vi "GoTo.vi"(6 "Busy":refnum<vi>, 8 "error in (no error)":errorcluster, 10 "Param":string, 11 "Controlador in":refnum<class "Controlador.lvclass">) -> (0 "error out":errorcluster, 2 "Response":string, 3 "Controlador out":refnum<class "Controlador.lvclass">)   [LabVIEW 2011]
uses:
  GLOBAL.vi
  Controlador.lvclass
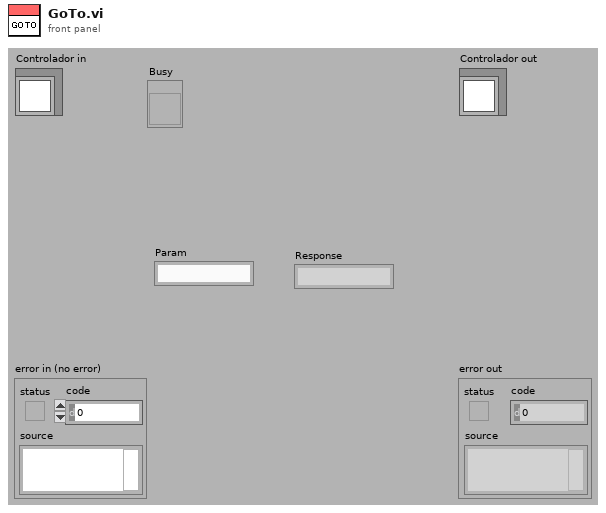
[diagram p1: front panel]
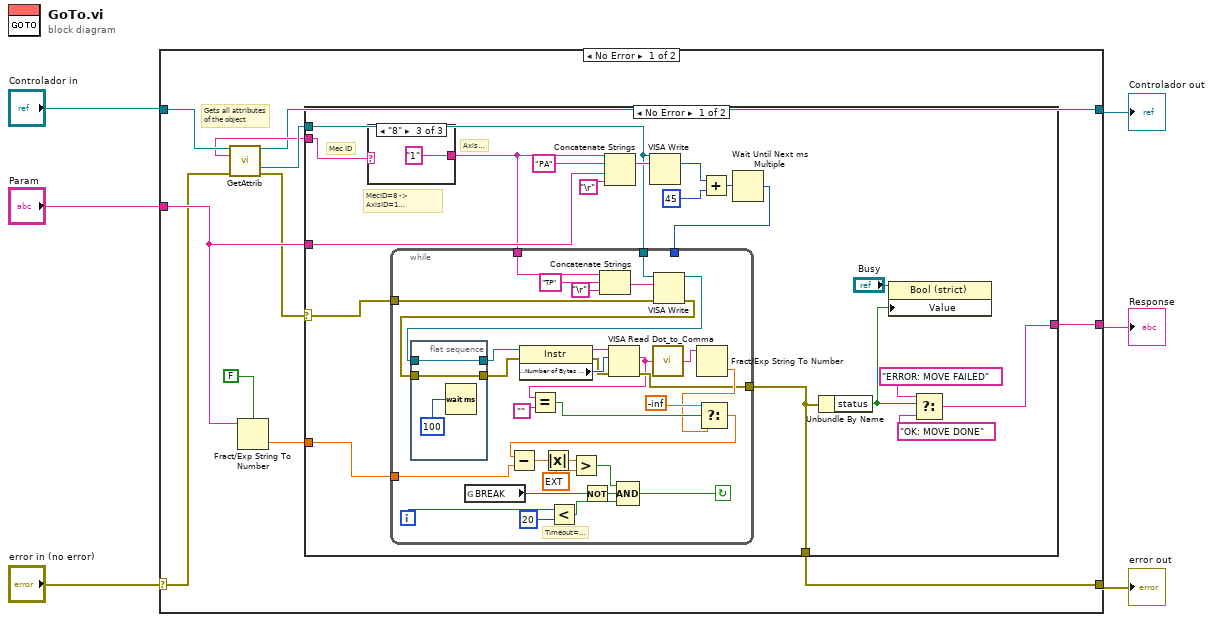
[diagram p0: block diagram]
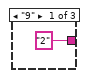
[diagram p2: hidden frame]
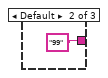
[diagram p3: hidden frame]
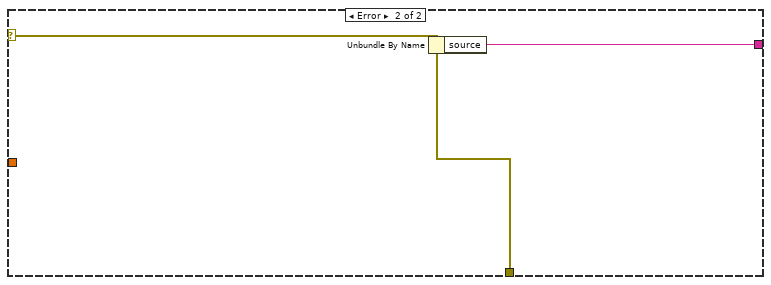
[diagram p4: hidden frame]
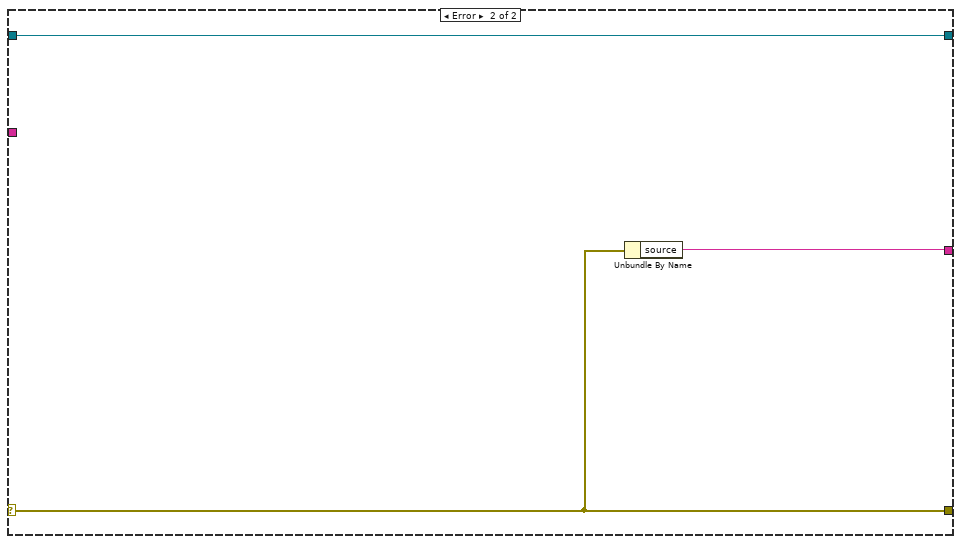
[diagram p5: hidden frame]
diagram:
  n1 = case shown="No Error" "error in (no error)" {
    selector: "error in (no error)" -> [w15 w78]
    tunnel: [w11 w79] -> w6
    tunnel: "Controlador in" -> [w14 w79]
    tunnel: [w10 w78] -> w2
    tunnel: "Param" -> [w17 _]
    tunnel: [w9 w77] -> w1
    frame No Error {
      # "Gets all attributes \nof the object"
      n2 = call "GetAttrib.vi"("Device in"=w14, "error in (no error)"=w15) -> ("Device out"=w11:refnum<class "Controlador.lvclass">, "Mec ID"=w12:string, "VISA Mec"=w13:refnum<visa-resource-name>, "error out"=w8:errorcluster)  [unwired: 10 out]
      n3 = Fract/Exp String To Number(use system decimal point (T)=FALSE, string=w17) -> (number=w16:dbl)  [unwired: 3 out]
      n4 = case shown="No Error" w8 {
        selector: w8 -> [w22 w76]
        tunnel: w17 -> [w29 _]
        tunnel: w16 -> [w28 _]
        tunnel: w13 -> [w27 _]
        tunnel: w12 -> [w18 _]
        tunnel: [w26 w76] -> w10
        tunnel: [w23 w75] -> w9
        frame No Error {
          # "MecID=8 -> AxisID=1\nMecID=9 -> AxisID=2"
          # "Axis ID"
          # "Mec ID"
          n5 = case shown="\"8\"" w18 {
            tunnel: ["2" "99" "1"] -> w19
            frame "9" {
            }
            frame Default {
            }
            frame "8" {
            }
          }
          n6 = Concatenate Strings(w19, "PA", w29, "\r") -> (w32:string)
          n7 = VISA Write(VISA resource name=w27, write buffer=w32) -> (return count=w33:u32)  [unwired: 1 in, 2 out]
          n8 = Add(x=w33, y=u32 45) -> (x+y=w35:u32)
          n9 = Wait Until Next ms Multiple(millisecond multiple=w35) -> (millisecond timer value=w36:u32)
          n10 = while {
            tunnel: w27 -> [w71]
            tunnel: w19 -> [w42]
            tunnel: w28 -> [w46]
            tunnel: w36 -> [_]
            tunnel: [w52] -> w26
            tunnel: w22 -> [w51]
            i -> [w45]
            stop <- w60 continue-if-true
            # "Timeout=2s"
            n11 = flat-sequence {
              tunnel: w50 -> [w74]
              tunnel: w49 -> [w73]
              tunnel: [w74] -> w48
              tunnel: [w73] -> w47
              frame #0 {
                n12 = Wait (ms)(milliseconds to wait=u32 100) -> ()  [unwired: 1 out]
              }
            }
            n13 = global read "GLOBAL.vi" "BREAK"() -> (w54:bool)
            n14 = property class="Instr"(reference=w47, error in=w48) -> (reference out=w68:refnum<visa-resource-name>, error out=w58:errorcluster, "Serial Settings:Number of Bytes at Serial Port"=w69:u32)
            n15 = Less?(x=w45, y=20) -> (x < y?=w43:bool)
            n16 = Not(x=w54) -> (.not. x?=w62:bool)
            n17 = Concatenate Strings(w42, "TP" ("string"), "\r") -> (w70:string)
            n18 = VISA Read(VISA resource name=w68, byte count=w69, error in (no error)=w58) -> (read buffer=w40:string, error out=w52:errorcluster)  [unwired: 2 out]
            n19 = Equal?(x=w40, y="") -> (x = y?=w55:bool)
            n20 = call "Dot_to_Comma.vi"("String in"=w40) -> ("String out"=w63:string)
            n21 = VISA Write(VISA resource name=w71, write buffer=w70, error in (no error)=w51) -> (VISA resource name out=w49:refnum<visa-resource-name>, error out=w50:errorcluster)  [unwired: 1 out]
            n22 = Fract/Exp String To Number(string=w63) -> (number=w53:dbl)  [unwired: 4 out]
            n23 = Select(t=-inf, s=w55, f=w53) -> (s? t:f=w57:dbl)
            n24 = Subtract(x=w57, y=w46) -> (x-y=w67:dbl)
            n25 = Absolute Value(x=w67) -> (abs(x)=w66:dbl)
            n26 = Greater?(x=w66, y=ext 0.03) -> (0:w61:bool)
            n27 = Compound Arithmetic op=AND(w61, w62, w43) -> (w60:bool)
          }
          n28 = Unbundle By Name(w26) -> ("status"=w20:bool)
          n29 = property class="Bool (strict)"(reference="Busy", "Value"=w20) -> ()  [unwired: 1 in, 2 out]
          n30 = Select(t="ERROR: MOVE FAILED", s=w20, f="OK: MOVE DONE") -> (s? t:f=w23:string)
        }
        frame Error {
          n31 = Unbundle By Name(w76) -> ("source"=w75:string)
        }
      }
    }
    frame Error {
      n32 = Unbundle By Name(w78) -> ("source"=w77:string)
    }
  }
  "error out" <- w2
  "Controlador out" <- w6
  "Response" <- w1
